vi "Write UI Ref Max F.vi"(8 "error in (no error)":errorcluster, 10 "UI Ref Max F":refnum<vi>, 11 "Analyze Results Fluence in":refnum<class "Analyze Results Fluence.lvclass">) -> (0 "error out":errorcluster, 3 "Analyze Results Fluence out":refnum<class "Analyze Results Fluence.lvclass">)   [LabVIEW 2014, in "Analyze Results Fluence.lvclass"]
uses:
  Analyze Results Fluence.lvclass
  Analyze Results Fluence.lvclass/Analyze Results Fluence.ctl
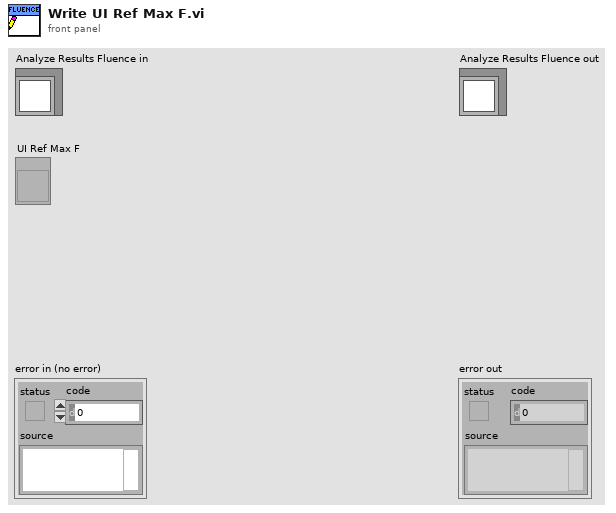
[diagram p1: front panel]
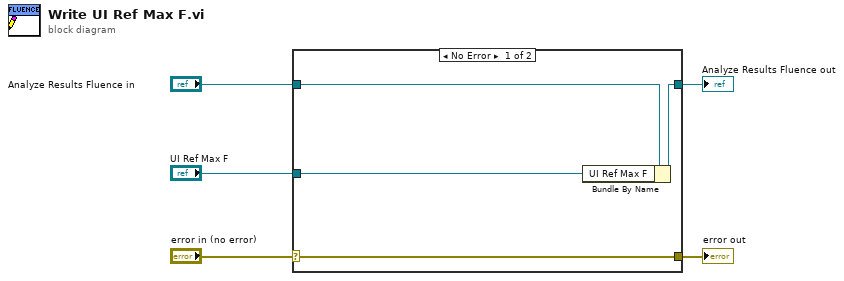
[diagram p0: block diagram]
diagram:
  n1 = case shown="No Error" "error in (no error)" {
    selector: "error in (no error)" -> [w9 w10]
    tunnel: [w9 w10] -> w4
    tunnel: [w7 w11] -> w2
    tunnel: "Analyze Results Fluence in" -> [w8 w11]
    tunnel: "UI Ref Max F" -> [w6 _]
    frame No Error {
      n2 = Bundle By Name(cluster=w8, "UI Ref Max F"=w6) -> (w7:refnum<class "Analyze Results Fluence.lvclass">)
    }
    frame Error {
    }
  }
  "error out" <- w4
  "Analyze Results Fluence out" <- w2
